vi "Mobility-Vt Calculator_Saturation_08_29_12a_JW.vi"(0 "Vg Column":dbl[](array[numeric]), 5 "Sat Id Column":dbl[](array[numeric]), 7 "NumPts":i32=5, 9 "Input Cluster":T1) -> (1 "Used Points":cluster{"Vg Used":dbl[], "Sqrt(Id) Used ":dbl[]}, 2 "Check Cluster":T2, 3 "Log Graph":cluster{dbl[], dbl[]}[](graph), 4 "Mobility-Sat":dbl format="%#_4e", 6 "VT-Sat":dbl, 8 "Index-Sat":i32, 10 "Sqrt Plot":cluster{dbl[], dbl[]}[](graph), 13 "Raw Graph":cluster{dbl[], dbl[]}[](graph), 14 "Off I-Sat":dbl format="%_6g", 15 "On/Off I-Sat":dbl)   [LabVIEW 2012]
uses:
  <vilib>/Analysis/NI_AALPro.lvlib
panel:
  out "Off I-Sat 2":dbl
  out "Capacitance (C)":dbl
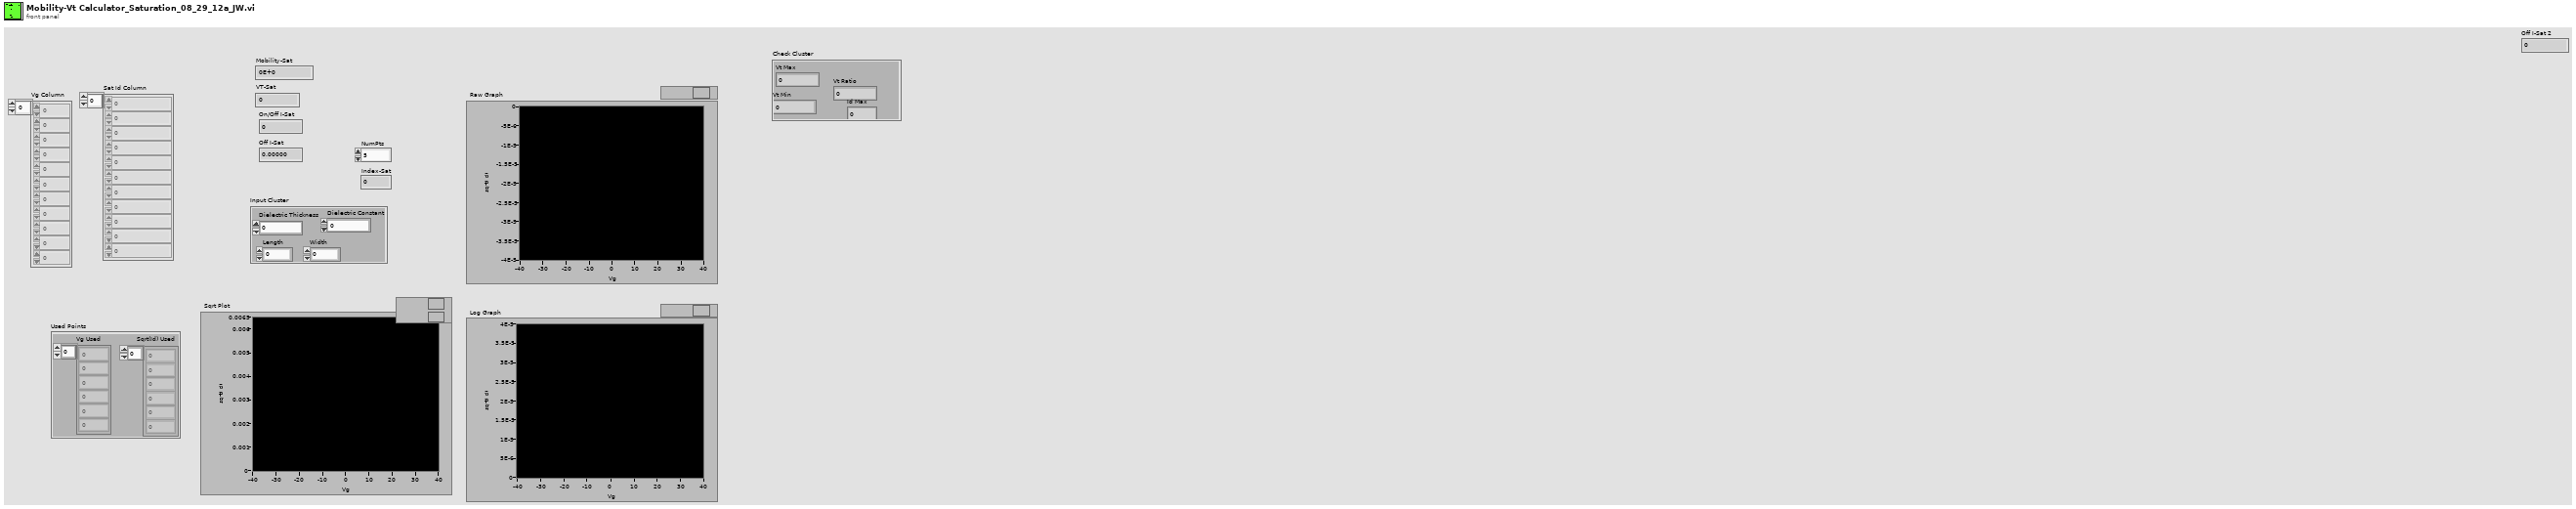
[diagram p1: front panel]
types:
  T1 = cluster{"Length":dbl, "Width":dbl, "Dielectric Thickness":dbl, "Dielectric Constant":dbl}
  T2 = cluster{"Vt Max":dbl, "Vt Min":dbl, "Vt Ratio":dbl, "Id Max":dbl}
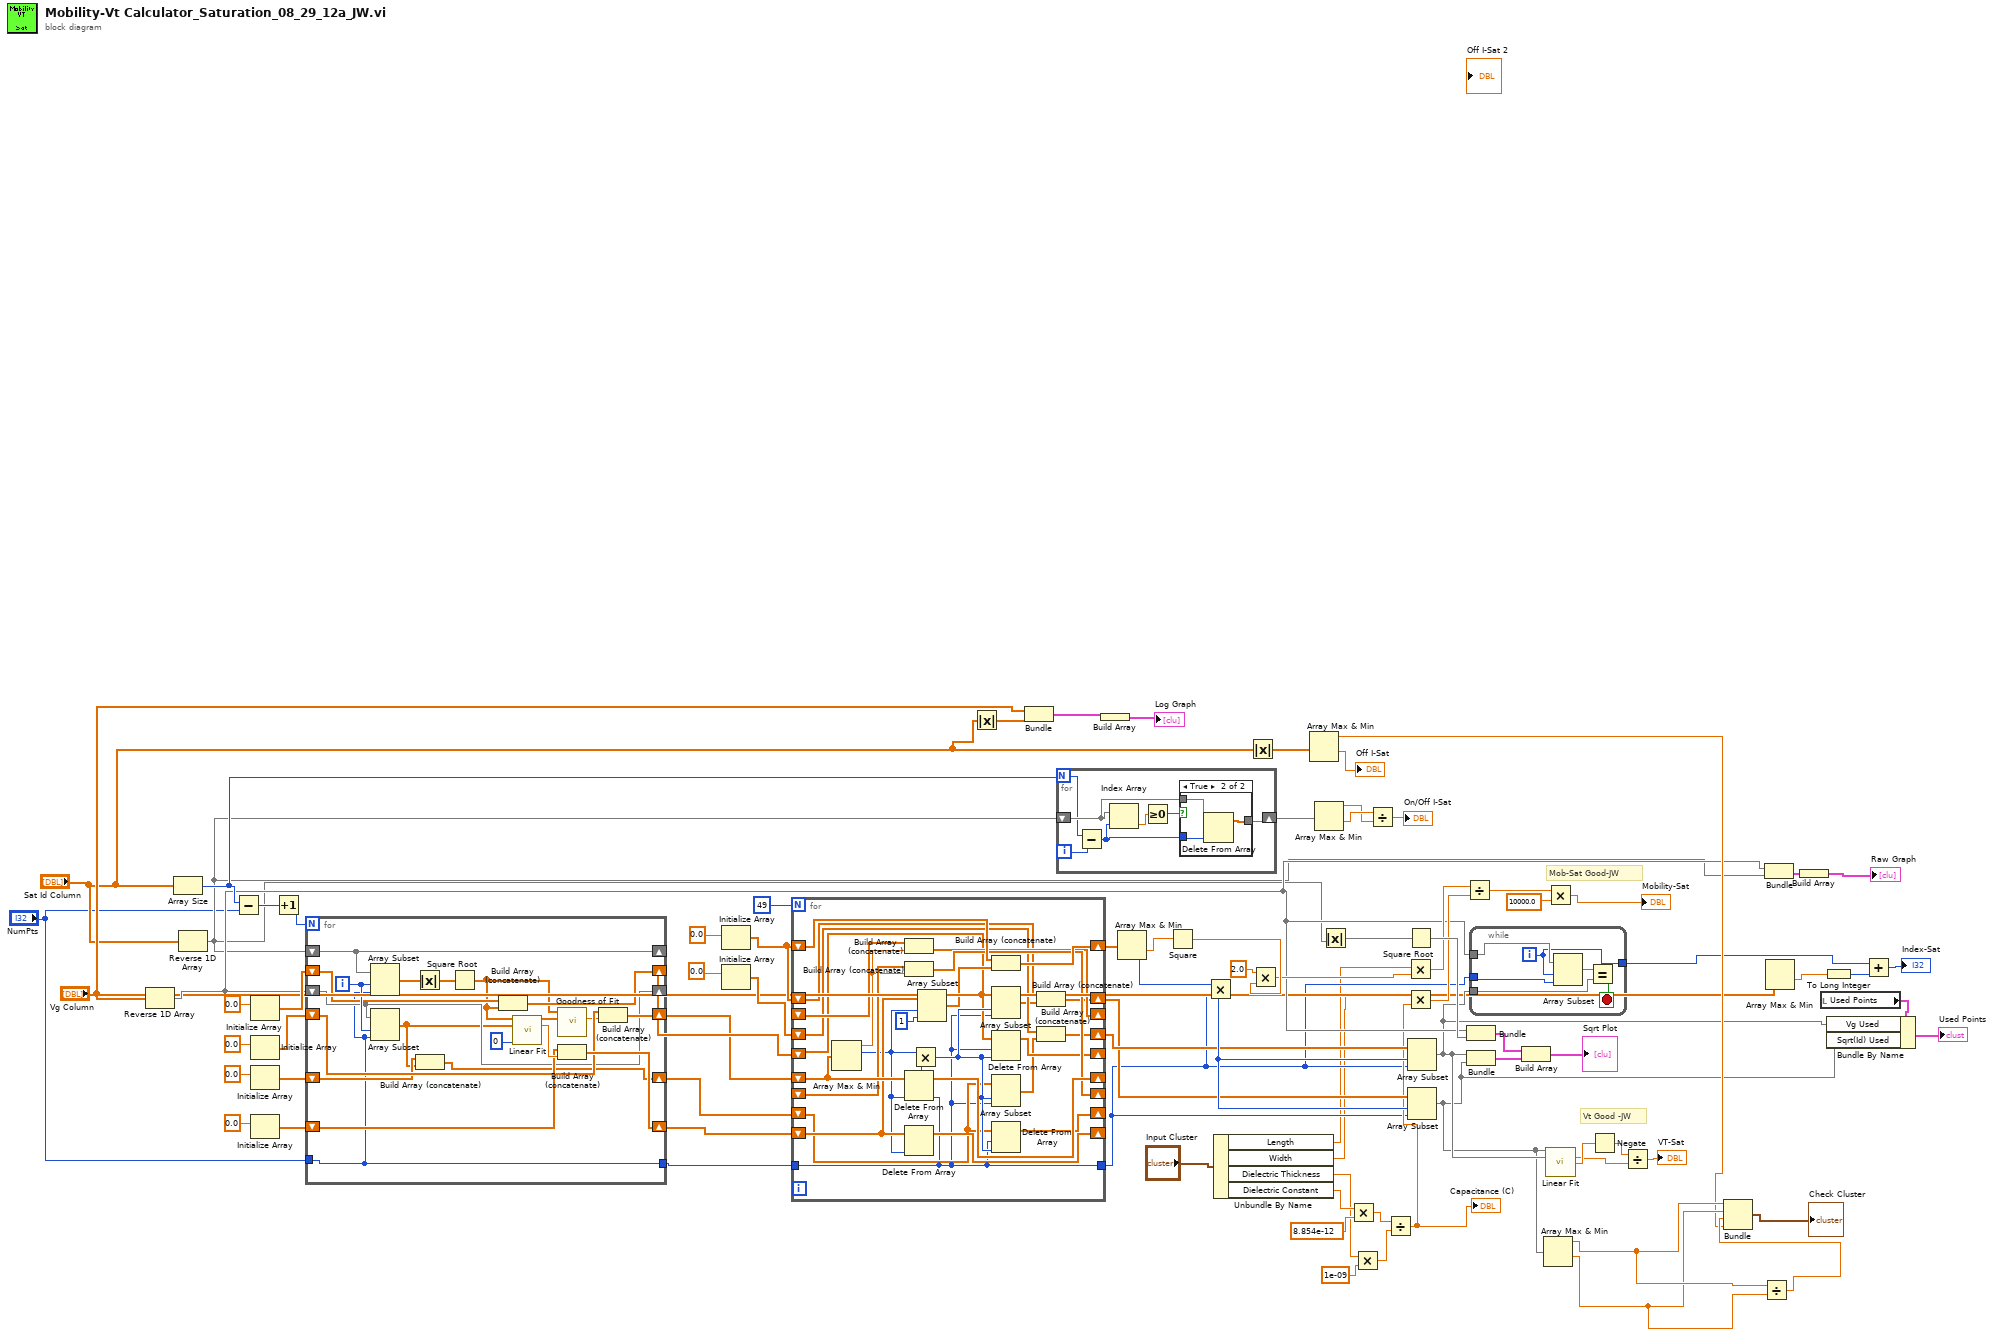
[diagram p0: block diagram]
diagram:
  # "Mob-Sat Good-JW"
  # "Vt Good -JW"
  n1 = Reverse 1D Array(array="Vg Column") -> (reversed array=w28:dbl[])
  n2 = Array Size(array="Sat Id Column") -> (size(s)=w38:i32)
  n3 = Reverse 1D Array(array="Sat Id Column") -> (reversed array=w27:dbl[])
  n4 = Subtract(x=w38, y="NumPts") -> (x-y=w82:i32)
  n5 = Initialize Array(0.0) -> (w69:dbl[])  [unwired: 1 in]
  n6 = Initialize Array(0.0) -> (w58:dbl[])  [unwired: 1 in]
  n7 = Initialize Array(0.0) -> (w70:dbl[])  [unwired: 1 in]
  n8 = Initialize Array(0.0) -> (w57:dbl[])  [unwired: 1 in]
  n9 = Increment(x=w82) -> (x+1=w83:i32)
  n10 = for {
    N: w83 -> [_]
    shift-right: [w90] -> _
    shift-left: w28 -> [w90]
    shift-right: [w98] -> _
    shift-left: w27 -> [w98]
    shift-right: [w102] -> w63
    shift-left: w57 -> [w101]
    shift-right: [w100] -> w65
    shift-left: w58 -> [w99]
    tunnel: "NumPts" -> [w85]
    shift-right: [w93] -> w71
    shift-left: w69 -> [w94]
    shift-right: [w91] -> w72
    shift-left: w70 -> [w92]
    tunnel: [w85] -> w7
    i -> [w104]
    n11 = Array Subset(array=w98, index=w104, length=w85) -> (w97:dbl[])
    n12 = Array Subset(array=w90, index=w104, length=w85) -> (w89:dbl[])
    n13 = Absolute Value(x=w97) -> (abs(x)=w96:dbl[])
    n14 = Build Array (concatenate)(w92, w89) -> (w91:dbl[])
    n15 = Square Root(x=w96) -> (sqrt(x)=w86:dbl[])
    n16 = Build Array (concatenate)(w94, w86) -> (w93:dbl[])
    n17 = call <vilib>:"Linear Fit.vi"("Y"=w86, "X"=w89, "method"=0) -> ("Best Linear Fit"=w88:dbl[], "slope"=w103:dbl)  [unwired: 8 in, 3 out]
    n18 = call <vilib>:"Goodness of Fit.vi"("Best Fit"=w88, "Y"=w86) -> ("R-square"=w87:dbl)  [unwired: 6 in, 3 out]
    n19 = Build Array (concatenate)(w101, w103) -> (w102:dbl[])
    n20 = Build Array (concatenate)(w99, w87) -> (w100:dbl[])
  }
  n21 = Initialize Array(0.0) -> (w78:dbl[])  [unwired: 1 in]
  n22 = Initialize Array(0.0) -> (w73:dbl[])  [unwired: 1 in]
  n23 = for {
    N: 49 -> [_]
    shift-right: [w129] -> _
    shift-left: w65 -> [w130]
    shift-right: [w110] -> _
    shift-left: w63 -> [w111]
    shift-right: [w126] -> w64
    shift-left: w78 -> [w125]
    shift-right: [w124] -> _
    shift-left: _ -> [w123]
    shift-right: [w122] -> _
    shift-left: _ -> [w121]
    shift-right: [w120] -> _
    shift-left: w71 -> [w107]
    shift-right: [w118] -> _
    shift-left: w72 -> [w106]
    tunnel: w7 -> [w105]
    shift-right: [w117] -> w75
    shift-left: w78 -> [w116]
    shift-right: [w115] -> w76
    shift-left: w73 -> [w114]
    tunnel: [w105] -> w6
    n24 = Array Max & Min(array=w130) -> (max value=w109:dbl, max index (indices)=w108:i32)  [unwired: 2 out]
    n25 = Build Array (concatenate)(w121, w109) -> (w122:dbl[])
    n26 = Build Array (concatenate)(w123, w109) -> (w124:dbl[])
    n27 = Delete From Array(array=w130, index=w108) -> (array with subset deleted=w129:dbl[])  [unwired: 1 in, 1 out]
    n28 = Delete From Array(array=w111, index=w108) -> (array with subset deleted=w110:dbl[])  [unwired: 1 in, 1 out]
    n29 = Multiply(x=w108, y=w105) -> (x*y=w119:i32)
    n30 = Array Subset(array=w111, index=w108, length=1) -> (w127:dbl[])
    n31 = Build Array (concatenate)(w125, w127) -> (w126:dbl[])
    n32 = Array Subset(array=w107, index=w119, length=w105) -> (w112:dbl[])
    n33 = Delete From Array(array=w107, length=w105, index=w119) -> (array with subset deleted=w120:dbl[])  [unwired: 1 out]
    n34 = Array Subset(array=w106, index=w119, length=w105) -> (w113:dbl[])
    n35 = Delete From Array(array=w106, length=w105, index=w119) -> (array with subset deleted=w118:dbl[])  [unwired: 1 out]
    n36 = Build Array (concatenate)(w116, w112) -> (w117:dbl[])
    n37 = Build Array (concatenate)(w114, w113) -> (w115:dbl[])
  }
  n38 = Absolute Value(x="Sat Id Column") -> (abs(x)=w26:dbl[])
  n39 = Bundle("Vg Column"="Vg Column", w26) -> (w25:cluster{"Vg Column":dbl[], dbl[]})  [unwired: 1 in]
  n40 = for {
    N: w38 -> [w133]
    shift-right: [w136] -> w41
    shift-left: w27 -> [w137]
    i -> [w132]
    n41 = Subtract(x=w133, y=w132) -> (x-y=w131:i32)
    n42 = Index Array(array=w137, index=w131) -> (element=w134:dbl)
    n43 = Greater Or Equal To 0?(x=w134) -> (x >= 0?=w135:bool)
    n44 = case shown="True" w135 {
      tunnel: w137 -> [w138 w141]
      tunnel: w131 -> [_ w139]
      tunnel: [w138 w140] -> w136
      frame False {
      }
      frame True {
        n45 = Delete From Array(array=w141, index=w139) -> (array with subset deleted=w140:dbl[])  [unwired: 1 in, 1 out]
      }
    }
  }
  n46 = Build Array(w25) -> (→"Log Graph":cluster{"Vg Column":dbl[], dbl[]}[])
  n47 = Array Max & Min(array=w64) -> (min value=w61:dbl, min index (indices)=w77:i32)  [unwired: 2 out]
  n48 = Square(x=w61) -> (x^2=w56:dbl)
  n49 = Multiply(x=w77, y=w6) -> (x*y=w79:i32)
  n50 = Unbundle By Name("Input Cluster") -> ("Length"=w2:dbl, "Width"=w1:dbl, "Dielectric Thickness"=w3:dbl, "Dielectric Constant"=w4:dbl)
  n51 = Absolute Value(x="Sat Id Column") -> (abs(x)=w37:dbl[])
  n52 = Multiply(x=2.0, y=w56) -> (x*y=w55:dbl)
  n53 = Array Max & Min(array=w37) -> (max value=w32:dbl, min value=→"Off I-Sat":dbl)  [unwired: 2 out]
  n54 = Array Max & Min(array=w41) -> (max value=w39:dbl, min value=w40:dbl)  [unwired: 2 out]
  n55 = Absolute Value(x=w27) -> (abs(x)=w67:dbl[])
  n56 = Multiply(x=w4, y=8.854e-12) -> (x*y=w42:dbl)
  n57 = Multiply(x=w3, y=1e-09) -> (x*y=w44:dbl)
  n58 = Divide(x=w40, y=w39) -> (x/y=→"On/Off I-Sat":dbl)
  n59 = Divide(x=w42, y=w44) -> (x/y=w13:dbl)
  "Capacitance (C)" <- w13
  n60 = Multiply(x=w2, y=w55) -> (x*y=w54:dbl)
  n61 = Multiply(x=w1, y=w13) -> (x*y=w53:dbl)
  n62 = Square Root(x=w67) -> (sqrt(x)=w81:dbl[])
  n63 = Array Subset(array=w76, index=w79, length=w6) -> (w19:dbl[])
  n64 = Array Subset(array=w75, index=w79, length=w6) -> (w18:dbl[])
  n65 = Divide(x=w54, y=w53) -> (x/y=w51:dbl)
  n66 = Bundle(w28, w81) -> (w31:cluster{dbl[], dbl[]})  [unwired: 1 in]
  n67 = Bundle(w19, w18) -> (w80:cluster{dbl[], dbl[]})  [unwired: 1 in]
  n68 = while {
    tunnel: w28 -> [w146]
    tunnel: w19 -> [w143]
    tunnel: [w144] -> w23
    tunnel: w6 -> [w142]
    i -> [w144]
    stop <- w147 stop-if-true
    n69 = Array Subset(array=w146, index=w144, length=w142) -> (w145:dbl[])
    n70 = Equal?(x=w145, y=w143) -> (x = y?=w147:bool)
  }
  n71 = Build Array(w31, w80) -> (→"Sqrt Plot":cluster{dbl[], dbl[]}[])
  n72 = Array Max & Min(array=w18) -> (max value=w36:dbl, min value=w35:dbl)  [unwired: 2 out]
  n73 = Multiply(x=w51, y=10000.0) -> (x*y=→"Mobility-Sat":dbl)
  n74 = call <vilib>:"Linear Fit.vi"("Y"=w18, "X"=w19) -> ("slope"=w47:dbl, "intercept"=w49:dbl)  [unwired: 9 in, 3 out]
  n75 = Negate(x=w49) -> (-x=w48:dbl)
  n76 = Divide(x=w48, y=w47) -> (x/y=→"VT-Sat":dbl)
  n77 = Divide(x=w36, y=w35) -> (x/y=w34:dbl)
  n78 = Bundle(w36, w35, w34, w32) -> (→"Check Cluster":cluster{dbl, dbl, dbl, dbl})  [unwired: 1 in]
  n79 = Bundle(w28, w27) -> (w30:cluster{dbl[], dbl[]})  [unwired: 1 in]
  n80 = Array Max & Min(array="Vg Column") -> (min value=w15:dbl)  [unwired: 3 out]
  n81 = Build Array(w30) -> (→"Raw Graph":cluster{dbl[], dbl[]}[])
  n82 = local read "Used Points"() -> (w21:cluster{"Vg Used":dbl[], "Sqrt(Id) Used ":dbl[]})
  n83 = To Long Integer(number=w15) -> (32bit integer=w14:i32)
  n84 = Bundle By Name(cluster=w21, "Vg Used"=w19, "Sqrt(Id) Used"=w18) -> (→"Used Points":cluster{"Vg Used":dbl[], "Sqrt(Id) Used ":dbl[]})
  n85 = Add(x=w23, y=w14) -> (x+y=→"Index-Sat":i32)
